vi "Open Log File.vi"(8 "error in (no error)":errorcluster, 10 "Path":path, 11 "Word Logger Interface in":refnum<class "Word Logger Interface.lvclass">) -> (0 "error out":errorcluster, 3 "Word Logger Interface out":refnum<class "Word Logger Interface.lvclass">)   [LabVIEW 2020, in "Ballard ARINC 429 Engine.lvlib" / "Implementation.lvlib" / "Word Logging.lvlib" / "Word Logger Interface.lvclass"]
uses:
  Word Logger Interface.lvclass
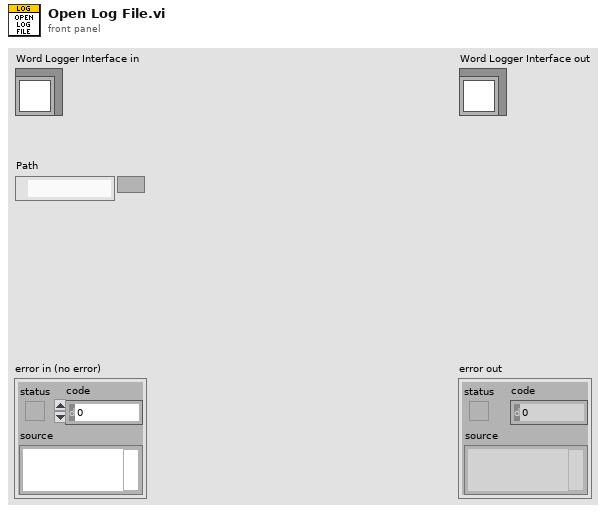
[diagram p1: front panel]
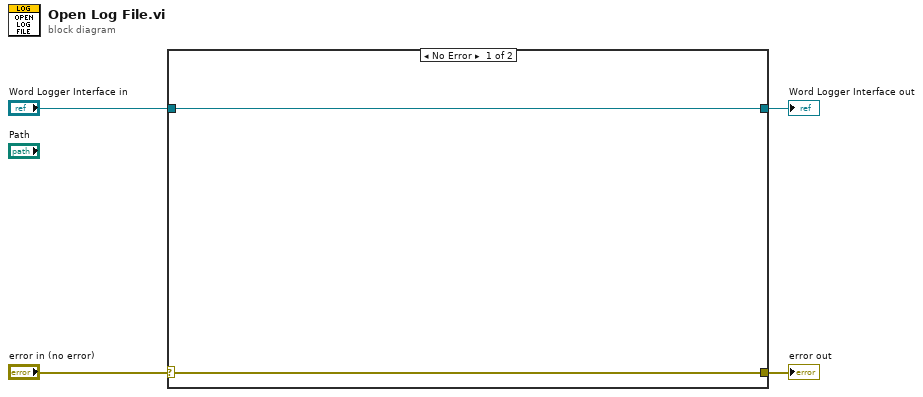
[diagram p0: block diagram]
diagram:
  n1 = case shown="No Error" "error in (no error)" {
    selector: "error in (no error)" -> [w5 w8]
    tunnel: [w5 w8] -> w3
    tunnel: [w6 w7] -> w1
    tunnel: "Word Logger Interface in" -> [w6 w7]
    frame No Error {
    }
    frame Error {
    }
  }
  "error out" <- w3
  "Word Logger Interface out" <- w1
